vi "AutoGenerate.vi"(8 "error in (no error)":errorcluster, 9 "GridData":string[][](array[string]), 10 "ColumnSetup":T1(array[cluster]) {"AutoSizeMode" items=["None"=1, "ColumnHeader"=2, "AllCellsExceptHeader"=4, "AllCells"=6, "DisplayedCellsExceptHeader"=8, "DisplayedCells"=10, "Fill"=16]}, 11 "DataGridView in":refnum<class "DataGridView.lvclass">) -> (0 "error out":errorcluster, 3 "DataGridView out":refnum<class "DataGridView.lvclass">)   [LabVIEW 2014, in "DataGridView.lvclass"]
uses:
  DataGridView.lvclass
  DataGridView.lvclass/DataGridView.ctl
  System.Data
  System.Windows.Forms
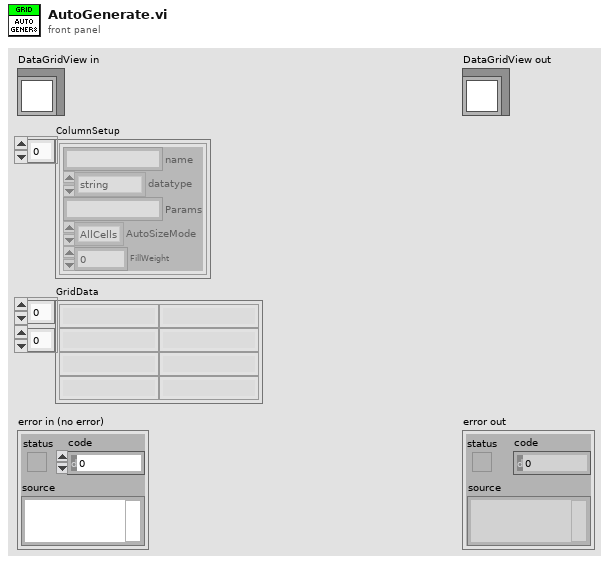
[diagram p1: front panel]
types:
  T1 = cluster{"name":string, "datatype":enum16{"string", "image", "check", "numeric", "timestamp"}, "Params":string, "AutoSizeMode":i32, "FillWeight":sgl}[]
  T2 = enum16{"string", "image", "check", "numeric", "timestamp"}
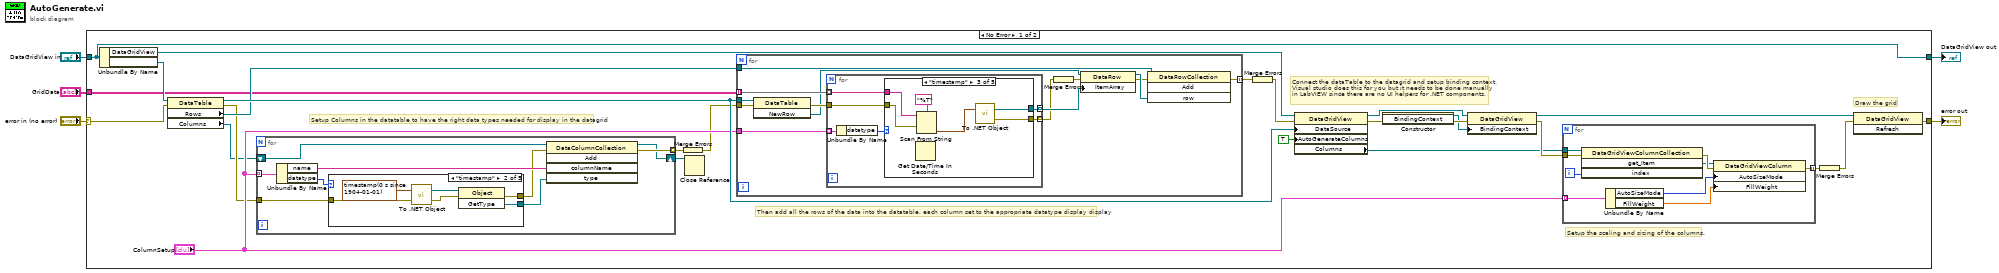
[diagram p0: block diagram]
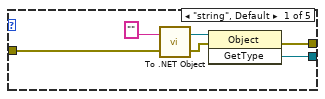
[diagram p2: hidden frame]
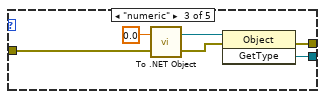
[diagram p3: hidden frame]
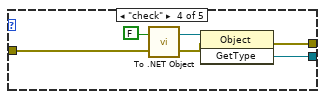
[diagram p4: hidden frame]
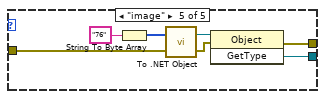
[diagram p5: hidden frame]
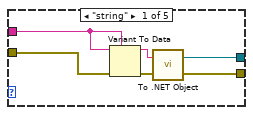
[diagram p6: hidden frame]
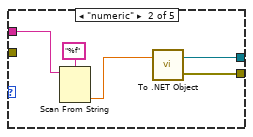
[diagram p7: hidden frame]
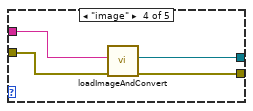
[diagram p8: hidden frame]
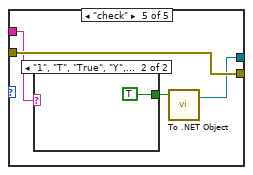
[diagram p9: hidden frame]
diagram:
  n1 = case shown="No Error" "error in (no error)" {
    selector: "error in (no error)" -> [w22 w127]
    tunnel: [w30 w127] -> w4
    tunnel: [w31 w126] -> w2
    tunnel: "DataGridView in" -> [w31 w126]
    tunnel: "GridData" -> [w20 _]
    frame No Error {
      # "Draw the grid"
      # "Setup the scaling and sizing of the columns."
      # "Connect the dataTable to the datagrid and setup binding context.\nVisual studio does this for you but it needs to be done manually\nin LabVIEW since there are no UI helpers for .NET components."
      # "Then add all the rows of the data into the datatable, each column set to the appropriate datatype display display"
      # "Setup Columns in the datatable to have the right data types needed for display in the datagrid"
      n2 = Unbundle By Name(w31) -> ("DataGridView"=w18:refnum<k24>, "DataTable"=w21:refnum<k24>)
      n3 = property class="DataTable"(reference=w21, error in=w22) -> (reference out=w24:refnum<k24>, error out=w14:errorcluster, "Rows"=w23:refnum<k24>, "Columns"=w7:refnum<k24>)
      n4 = for {
        tunnel: "ColumnSetup" -> [w48] mode=indexing
        tunnel: w14 -> [w43]
        tunnel: [w47] -> w16 mode=indexing
        shift-right: [w41] -> w6
        shift-left: w7 -> [w49]
        n5 = Unbundle By Name(w48) -> ("name"=w46:string, "datatype"=w44:T2)
        n6 = case shown="\"timestamp\"" w44 {
          tunnel: [w53 w59 w62 w71 w77] -> w45
          tunnel: w43 -> [w50 w56 w63 w68 w75]
          tunnel: [w52 w57 w64 w70 w74] -> w42
          frame "string", Default {
            n7 = call <vilib>:"To .NET Object.vi"("error in (no error)"=w50, "anything"="" ("name")) -> ("error out"=w51:errorcluster, ".NET object"=w54:refnum<k24>)
            n8 = invoke class="Object" method="GetType"(reference=w54, error in=w51) -> (error out=w52:errorcluster, "GetType"=w53:refnum<k24>)  [unwired: 1 in, 1 out]
          }
          frame "timestamp" {
            n9 = call <vilib>:"To .NET Object.vi"("error in (no error)"=w56, "anything"=timestamp(0 s since 1904-01-01) ("name")) -> ("error out"=w58:errorcluster, ".NET object"=w60:refnum<k24>)
            n10 = invoke class="Object" method="GetType"(reference=w60, error in=w58) -> (error out=w57:errorcluster, "GetType"=w59:refnum<k24>)  [unwired: 1 in, 1 out]
          }
          frame "numeric" {
            n11 = call <vilib>:"To .NET Object.vi"("error in (no error)"=w63, "anything"=0.0 ("name")) -> ("error out"=w65:errorcluster, ".NET object"=w66:refnum<k24>)
            n12 = invoke class="Object" method="GetType"(reference=w66, error in=w65) -> (error out=w64:errorcluster, "GetType"=w62:refnum<k24>)  [unwired: 1 in, 1 out]
          }
          frame "check" {
            n13 = call <vilib>:"To .NET Object.vi"("error in (no error)"=w68, "anything"=FALSE) -> ("error out"=w69:errorcluster, ".NET object"=w73:refnum<k24>)
            n14 = invoke class="Object" method="GetType"(reference=w73, error in=w69) -> (error out=w70:errorcluster, "GetType"=w71:refnum<k24>)  [unwired: 1 in, 1 out]
          }
          frame "image" {
            n15 = String To Byte Array(string="76") -> (unsigned byte array=w79:u8[])
            n16 = call <vilib>:"To .NET Object.vi"("error in (no error)"=w75, "anything"=w79) -> ("error out"=w76:errorcluster, ".NET object"=w80:refnum<k24>)
            n17 = invoke class="Object" method="GetType"(reference=w80, error in=w76) -> (error out=w74:errorcluster, "GetType"=w77:refnum<k24>)  [unwired: 1 in, 1 out]
          }
        }
        n18 = invoke class="DataColumnCollection" method="Add"(reference=w49, error in=w42, "columnName"=w46, "type"=w45) -> (reference out=w41:refnum<k24>, error out=w47:errorcluster)  [unwired: 1 in, 3 out]
      }
      n19 = Merge Errors(w16) -> (w9:errorcluster)
      n20 = Close Reference(reference=w6) -> ()  [unwired: 1 in, 1 out]
      n21 = for {
        tunnel: w23 -> [w92]
        tunnel: w24 -> [w93]
        tunnel: [w91] -> w25 mode=indexing
        tunnel: w20 -> [w90] mode=indexing
        tunnel: "ColumnSetup" -> [w82]
        tunnel: w9 -> [w81]
        n22 = invoke class="DataTable" method="NewRow"(reference=w93, error in=w81) -> (error out=w89:errorcluster, "NewRow"=w88:refnum<k24>)  [unwired: 1 in, 1 out]
        n23 = for {
          tunnel: w90 -> [w99] mode=indexing
          tunnel: [w98] -> w86 mode=indexing
          tunnel: w89 -> [w97]
          tunnel: [w96] -> w85 mode=indexing
          tunnel: w82 -> [w95] mode=indexing
          n24 = Unbundle By Name(w95) -> ("datatype"=w94:T2)
          n25 = case shown="\"timestamp\"" w94 {
            tunnel: w99 -> [w101 w108 w114 w120 w122]
            tunnel: [w100 w109 w115 w119 w123] -> w98
            tunnel: w97 -> [w104 _ w112 w118 w124]
            tunnel: [w102 w110 w116 w117 w124] -> w96
            frame "string" {
              n26 = Variant To Data(error in=w104, type=w101, Variant=w101) -> (data=w105:string, error out=w103:errorcluster)
              n27 = call <vilib>:"To .NET Object.vi"("error in (no error)"=w103, "anything"=w105) -> ("error out"=w102:errorcluster, ".NET object"=w100:refnum<k24>)
            }
            frame "numeric" {
              n28 = Scan From String(format string="%f", input string=w108) -> (output 1=w106:dbl)  [unwired: 3 in, 3 out]
              n29 = call <vilib>:"To .NET Object.vi"("anything"=w106) -> ("error out"=w110:errorcluster, ".NET object"=w109:refnum<k24>)  [unwired: 1 in]
            }
            frame "timestamp" {
              n30 = Get Date/Time In Seconds() -> ()  [unwired: 1 out]
              n31 = Scan From String(format string="%T", input string=w114, error in=w112) -> (output 1=w111:timestamp)  [unwired: 2 in, 3 out]
              n32 = call <vilib>:"To .NET Object.vi"("anything"=w111) -> ("error out"=w116:errorcluster, ".NET object"=w115:refnum<k24>)  [unwired: 1 in]
            }
            frame "image" {
              n33 = call "loadImageAndConvert.vi"("error in (no error)"=w118, "name or relative path"=w120) -> ("error out"=w117:errorcluster, ".NET object"=w119:refnum<k24>)  [unwired: 8 in]
            }
            frame "check" {
              n34 = case shown="\"1\", \"T\", \"True\", \"Y\", \"Yes\"" w122 {
                tunnel: [_ TRUE] -> w121
                frame Default {
                }
                frame "1", "T", "True", "Y", "Yes" {
                }
              }
              n35 = call <vilib>:"To .NET Object.vi"("anything"=w121) -> (".NET object"=w123:refnum<k24>)  [unwired: 1 in, 1 out]
            }
          }
        }
        n36 = Merge Errors(w85) -> (w84:errorcluster)
        n37 = property class="DataRow"(reference=w88, error in=w84, "ItemArray"=w86) -> (reference out=w87:refnum<k24>, error out=w83:errorcluster)
        n38 = invoke class="DataRowCollection" method="Add"(reference=w92, error in=w83, "row"=w87) -> (error out=w91:errorcluster)  [unwired: 1 in, 3 out]
      }
      n39 = Merge Errors(w25) -> (w15:errorcluster)
      n40 = property class="DataGridView"(reference=w18, error in=w15, "DataSource"=w24, "AutoGenerateColumns"=TRUE) -> (reference out=w13:refnum<k24>, error out=w26:errorcluster, "Columns"=w8:refnum<k24>)
      n41 = constructor class="BindingContext"(error in=w26) -> (reference out=w28:refnum<k24>, error out=w29:errorcluster)  [unwired: 2 in, 1 out]
      n42 = property class="DataGridView"(reference=w13, error in=w29, "BindingContext"=w28) -> (reference out=w27:refnum<k24>, error out=w12:errorcluster)
      n43 = for {
        tunnel: w8 -> [w36]
        tunnel: "ColumnSetup" -> [w40] mode=indexing
        tunnel: w12 -> [w35]
        tunnel: [w37] -> w11 mode=indexing
        i -> [w32]
        n44 = invoke class="DataGridViewColumnCollection" method="get_Item"(reference=w36, error in=w35, "index"=w32) -> (error out=w34:errorcluster, "get_Item"=w33:refnum<k24>)  [unwired: 1 in, 2 out]
        n45 = Unbundle By Name(w40) -> ("AutoSizeMode"=w39:i32, "FillWeight"=w38:sgl)
        n46 = property class="DataGridViewColumn"(reference=w33, error in=w34, "AutoSizeMode"=w39, "FillWeight"=w38) -> (error out=w37:errorcluster)  [unwired: 1 out]
      }
      n47 = Merge Errors(w11) -> (w10:errorcluster)
      n48 = invoke class="DataGridView" method="Refresh"(reference=w27, error in=w10) -> (error out=w30:errorcluster)  [unwired: 1 in, 2 out]
    }
    frame Error {
    }
  }
  "error out" <- w4
  "DataGridView out" <- w2
